vi "DAQAnalogTask.vi"() -> (0 "error out":errorcluster, 1 "Expected Signal Read":bool, 2 "Waveform Graph":waveform(dbl)(graph))   [LabVIEW 2011]
uses:
  <vilib>/DAQmx/read.llb/DAQmx Read (Analog Wfm 1Chan NSamp).vi
  Instance           1 21Saved   DAQAnalogTask .vi
  <vilib>/DAQmx/miscellaneous.llb/DAQmx Fill In Error Info.vi
panel:
  in  "Exprected Data":waveform(dbl)={"t0"=timestamp(3221915899.1693745 s since 1904-01-01), "dt"=0.001, "Y"=[0.01251220703125, 0.7733154296875, 1.119384765625, 1.748046875, 2.49420166015625, 3.06793212890625, 3.55926513671875, 4.1851806640625, 4.9346923828125, 5.2777099609375, 5.771484375, 6.26129150390625, 6.9744873046875, 7.16339111328125, 7.5689697265625, 7.95745849609375, 8.39385986328125, 8.88702392578125, 9.017333984375, 9.27703857421875, 9.64385986328125, 9.78668212890625, 9.832763671875, 9.920654296875, 9.9798583984375, 9.99969482421875, 9.9798583984375, 9.920654296875, 9.83001708984375, 9.82177734375, 9.47967529296875, 9.21966552734375, 9.073486328125, 8.68927001953125, 8.4979248046875, 8.2232666015625, 7.685546875, 7.40631103515625, 6.6973876953125, 6.50604248046875, 5.90789794921875, 5.4437255859375, 4.840087890625, 4.150390625, 3.59771728515625, 3.0548095703125, 2.33795166015625, 1.84906005859375, 1.1279296875, 0.6756591796875, 0.10650634765625, -0.75836181640625, -1.15997314453125, -1.824951171875, -2.42919921875, -2.999267578125, -3.671875, -4.20196533203125, -4.92431640625, -5.30120849609375, -5.80902099609375, -6.29058837890625, -6.98577880859375, -7.17864990234375, -7.66143798828125, -8.0279541015625, -8.56719970703125, -8.7469482421875, -8.91357421875, -9.42962646484375, -9.57763671875, -9.7918701171875, -9.67803955078125, -9.8846435546875, -9.9798583984375, -9.99969482421875, -9.9798583984375, -9.86236572265625, -9.90692138671875, -9.78851318359375, -9.5880126953125, -9.290771484375, -8.92730712890625, -8.880615234375, -8.3221435546875, -8.1072998046875, -7.830810546875, -7.20458984375, -6.94366455078125, -6.231689453125, -5.794677734375, -5.24688720703125, -4.9041748046875, -4.2706298828125, -3.8299560546875, -3.01483154296875, -2.6025390625, -1.90216064453125, -1.309814453125, -0.48004150390625], "attributes"=variant("NI_ChannelName"=variant(string "Voltage"), "NI_UnitDescription"=variant(string "Volts"))}
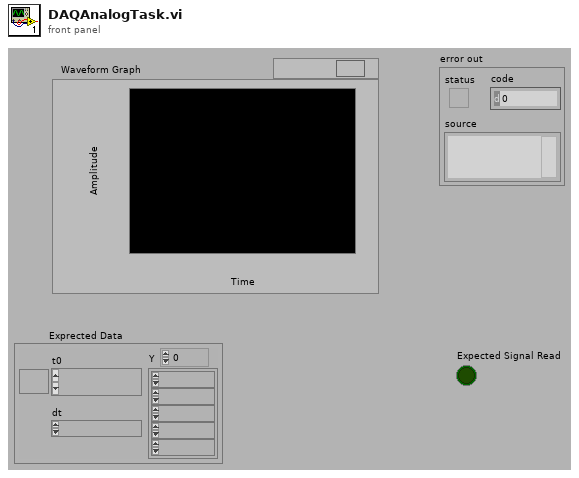
[diagram p1: front panel]
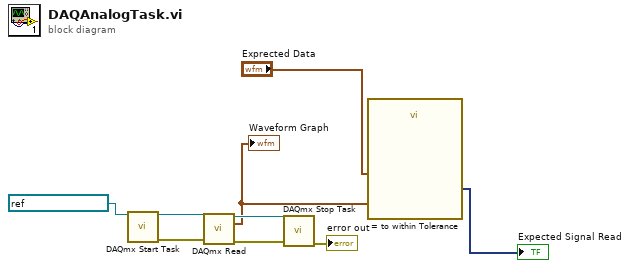
[diagram p0: block diagram]
diagram:
  n1 = call <vilib>:"DAQmx Start Task.vi"("task/channels in"=refnum<k21> "MyVoltageTask") -> ("task out"=w8:refnum<k21>, "error out"=w7:errorcluster)  [unwired: 13 in]
  n2 = call-poly <vilib>:"DAQmx Read.vi"("task/channels in"=w8, "error in"=w7) -> ("task out"=w5:refnum<k21>, "data"=w3:waveform(dbl), "error out"=w6:errorcluster)  [unwired: 11 in]
  "Waveform Graph" <- w3
  n3 = call <vilib>:"DAQmx Stop Task.vi"("task/channels in"=w5, "error in"=w6) -> ("error out"=→"error out":errorcluster)  [unwired: 12 in, 1 out]
  n4 = call "= to within Tolerance"("Operand 2"=w3, "Operand 1"="Exprected Data") -> ("Result"=→"Expected Signal Read":dynamicdata)  [unwired: 8 in, 1 out]
